vi "Submit.vi"(0 "Compound_Installer In":refnum<class "Compound_Installer.lvclass">) -> (4 "Compound_Installer Out":refnum<class "Compound_Installer.lvclass">)   [LabVIEW 2017, in "CL_G3_VIComponentBuilder.lvlib" / "Compound_Installer.lvclass"]
doc: "Invokes the commit behaivor specified by this export and any additional operations deemed necessary by the export."
uses:
  Compound_Installer.lvclass
  C:/Tool Chain Support/Software Module Builder/Source/Exports/Exports/Export.lvclass
  Compound_Installer.lvclass/Compound_Installer.ctl
  Exports/Export.lvclass/Export.ctl
  Exports/Accessors/Read Export Operation Errors.vi
  Accessors/Read Sub Export Build Order.vi
  Exports/Accessors/Write Export Operation Errors.vi
  Exports/Export.lvclass
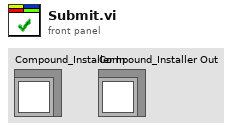
[diagram p1: front panel]
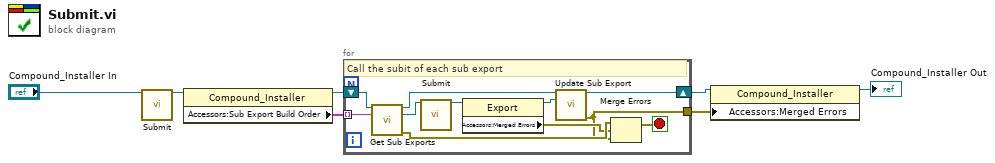
[diagram p0: block diagram]
diagram:
  n1 = call-parent "Submit.vi"("Export In"="Compound_Installer In") -> ("Export Out"=w6:refnum<class "Compound_Installer.lvclass">)  [unwired: 14 in]
  n2 = property class="Compound_Installer"(reference=w6) -> (reference out=w4:refnum<class "Compound_Installer.lvclass">, "Accessors:Sub Export Build Order"=w5:string[])  [unwired: 1 in, 1 out]
  n3 = for {
    tunnel: w5 -> [w18] mode=indexing
    shift-right: [w14] -> w3
    shift-left: w4 -> [w17]
    tunnel: [w8] -> w1
    stop <- w9 stop-if-true
    # "Call the subit of each sub export"
    n4 = call-dynamic "Get Sub Exports.vi"("NSIS_Installer in"=w17, "Sub Installer Name"=w18) -> ("NSIS_Installer out"=w16:refnum<class "Compound_Installer.lvclass">, "Export"=w15:refnum<class "Export.lvclass">, "error out"=w11:errorcluster)  [unwired: 10 in, 1 out]
    n5 = call-dynamic "Submit.vi"("Export In"=w15) -> ("Export Out"=w13:refnum<class "Export.lvclass">)  [unwired: 14 in]
    n6 = property class="Export"(reference=w13) -> (reference out=w12:refnum<class "Export.lvclass">, "Accessors:Merged Errors"=w10:errorcluster)  [unwired: 1 in, 1 out]
    n7 = call-dynamic "Update Sub Export.vi"("NSIS_Installer in"=w16, "Sub Export"=w12) -> ("NSIS_Installer out"=w14:refnum<class "Compound_Installer.lvclass">, "error out"=w8:errorcluster)  [unwired: 12 in]
    n8 = Merge Errors(w11, w10, w8) -> (w9:errorcluster)
  }
  n9 = property class="Compound_Installer"(reference=w3, "Accessors:Merged Errors"=w1) -> (reference out=→"Compound_Installer Out":refnum<class "Compound_Installer.lvclass">)  [unwired: 1 in, 1 out]
